vi "RS-xxx Factory.vi"(8 "error in (no error)":errorcluster, 10 "RS-xxx settings":T1={"Port"="", "Baud Rate"=0, "Data Bits"=0, "Parity"=enum."None", "Stop Bits"=0, "Flow Control"=0, "XON"=enum."NUL", "XOFF"=enum."NUL", "End Read on Termination Character"=FALSE, "End Write on Termination Character"=FALSE, "Termination Character"=0, "4wireMode"=TRUE, "AssertDTR"=TRUE, "WireMode"=-1} {"WireMode" items=["Unknown"=-1, "RS485/Wire4"=0, "RS485/Wire2-EchoDTR"=1, "RS485/Wire2-CtrlDTR"=2, "RS485/Wire2-Auto"=3, "RS232/DTE"=128, "RS232/DCE"=129, "RS232/Auto"=130]; "Baud Rate" items=["75", "110", "134", "150", "300", "600", "1200", "1800", "2400", "4800", "7200", "9600", "14400", "19200", "28800", "38400", "56000", "57600", "115200", "128000", "230400", "460800", "921600", "1843200", "3000000"]; "Stop Bits" items=["1", "1.5", "2"]}) -> (0 "error out":errorcluster, 3 "protocol out":refnum<class "Protocol Parent.lvclass">)   [LabVIEW 2023, in "Protocols.lvlib" / "RS-xxx.lvclass"]
doc: "Instantiate a new RS-xxx Protocol object using the provided RS-xxx Port settings."
uses:
  RS-xxx.lvclass
  Protocol Parent/Protocol Parent.lvclass
  RS-xxx Settings.ctl
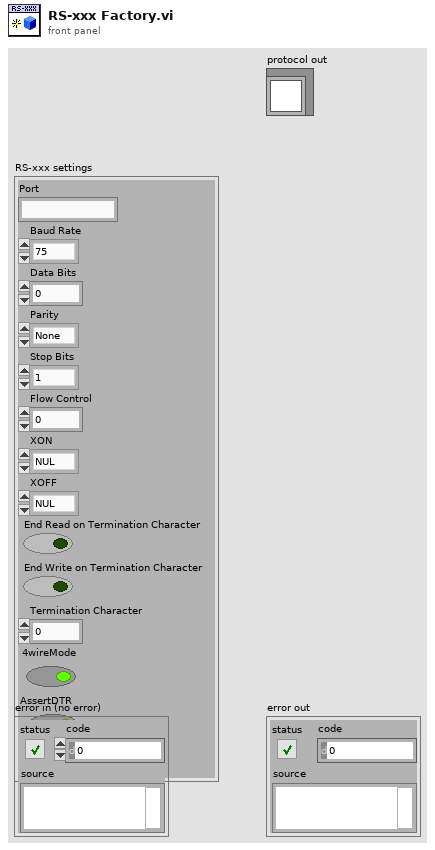
[diagram p1: front panel]
types:
  T1 = typedef "Protocols.lvlib/RS-xxx.lvclass/RS-xxx Settings.ctl" = cluster{"Port":string, "Baud Rate":u32, "Data Bits":u16, "Parity":enum16{"None", "Odd", "Even", "Mark", "Space"}, "Stop Bits":u16, "Flow Control":u16, "XON":enum16{"NUL", "SOH", "STX", "ETX", "EOT", "ENQ", "ACK", "BEL", "BS", "HT", "LF", "VT", "FF", "CR", "SO", "SI", "DLE", "DC1", "DC2", "DC3", "DC4", "NAK", "SYN", "ETB", "CAN", "EM", "SUB", "ESC", "FS", "GS", "RS", "US", "SP", "!", "\"", "#", "$", "%", "&", "'", "(", ")", "*", "+", ",", "- (-)", ".", "/", "0", "1", "2", "3", "4", "5", "6", "7", "8", "9", ":", ";", "<", "=", ">", "?", "@", "A", "B", "C", "D", "E", "F", "G", "H", "I", "J", "K", "L", "M", "N", "O", "P", "Q", "R", "S", "T", "U", "V", "W", "X", "Y", "Z", "[", "\\", "]", "^", "_", "`", "a", "b", "c", "d", "e", "f", "g", "h", "i", "j", "k", "l", "m", "n", "o", "p", "q", "r", "s", "t", "u", "v", "w", "x", "y", "z", "{", "|", "}", "~"}, "XOFF":enum16{"NUL", "SOH", "STX", "ETX", "EOT", "ENQ", "ACK", "BEL", "BS", "HT", "LF", "VT", "FF", "CR", "SO", "SI", "DLE", "DC1", "DC2", "DC3", "DC4", "NAK", "SYN", "ETB", "CAN", "EM", "SUB", "ESC", "FS", "GS", "RS", "US", "SP", "!", "\"", "#", "$", "%", "&", "'", "(", ")", "*", "+", ",", "- (-)", ".", "/", "0", "1", "2", "3", "4", "5", "6", "7", "8", "9", ":", ";", "<", "=", ">", "?", "@", "A", "B", "C", "D", "E", "F", "G", "H", "I", "J", "K", "L", "M", "N", "O", "P", "Q", "R", "S", "T", "U", "V", "W", "X", "Y", "Z", "[", "\\", "]", "^", "_", "`", "a", "b", "c", "d", "e", "f", "g", "h", "i", "j", "k", "l", "m", "n", "o", "p", "q", "r", "s", "t", "u", "v", "w", "x", "y", "z", "{", "|", "}", "~"}, "End Read on Termination Character":bool, "End Write on Termination Character":bool, "Termination Character":u8, "4wireMode":bool, "AssertDTR":bool, "WireMode":i16}
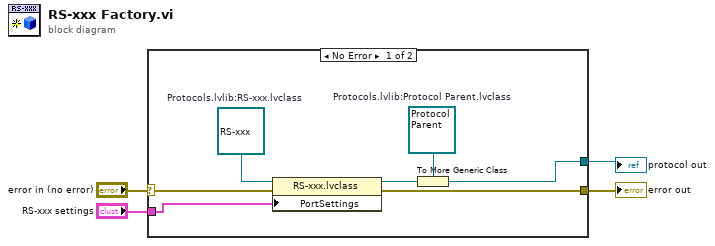
[diagram p0: block diagram]
diagram:
  n1 = case shown="No Error" "error in (no error)" {
    selector: "error in (no error)" -> [w8 w12]
    tunnel: "RS-xxx settings" -> [w10 _]
    tunnel: [w5 _] -> w1
    tunnel: [w9 w12] -> w3
    frame No Error {
      w6 = refnum<class "Protocol Parent.lvclass"> refnum  # Protocols.lvlib:Protocol Parent.lvclass
      w11 = refnum<class "RS-xxx.lvclass"> refnum  # Protocols.lvlib:RS-xxx.lvclass
      n2 = property class="RS-xxx.lvclass"(reference=w11, error in=w8, "PortSettings"=w10) -> (reference out=w7:refnum<class "RS-xxx.lvclass">, error out=w9:errorcluster)
      n3 = To More Generic Class(target class=w6, reference=w7) -> (generic class reference=w5:refnum<class "Protocol Parent.lvclass">)
    }
    frame Error {
    }
  }
  "error out" <- w3
  "protocol out" <- w1
